vi "Update_Attribute_Tree_POLARIS.vi"(4 "Flush Tree?":bool, 5 "error in":errorcluster, 6 "Filter":string, 7 "Tree Control In":refnum<vi>, 8 "Camera Name In":T1 caption="Session In") -> (0 "error out":errorcluster, 2 "Tree Control Out":refnum<vi>, 3 "Session Out":T1)   [LabVIEW 2014]
doc: "The Update Attribute Tree subVI, enumerates the attributes available for the camera and populates the Attribute Tree control with the attribute list."
uses:
  <vilib>/userdefined/High Color/IMAQdx.ctl
  <vilib>/vision/driver/NI_Vision_Acquisition_Software.lvlib
  <resource>/objmgr/imaqdx.rc
panel:
  out "ValuesArray":string[](array[string])
  out "AttibuteArray":string[](array[string])
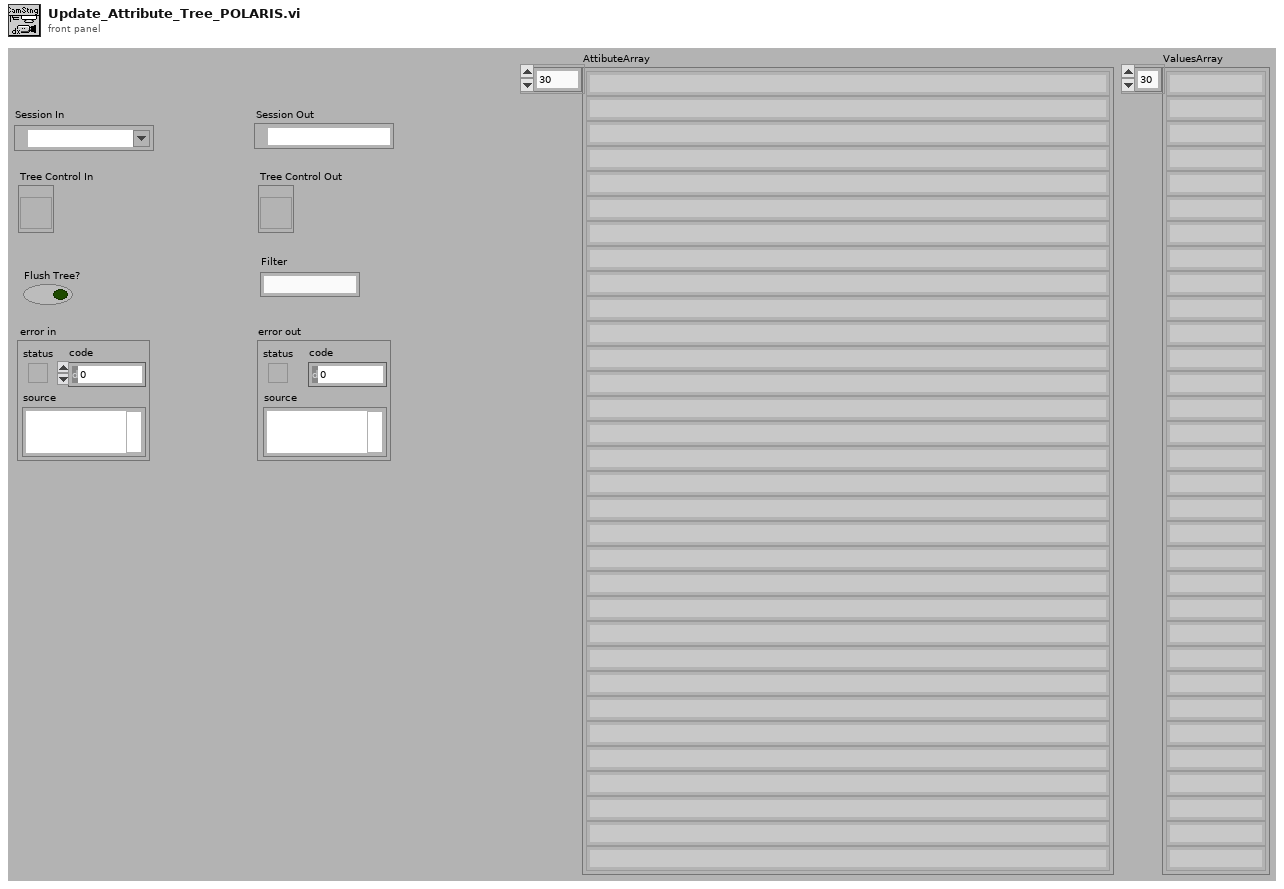
[diagram p1: front panel]
types:
  T1 = typedef "IMAQdx.ctl" = refnum<k21>
  T2 = typedef "NI_Vision_Acquisition_Software.lvlib/IMAQdx Attribute Type.ctl" = enum32{"U32", "I64", "DBL", "String", "Enum", "Bool", "Command"}
  T3 = cluster{"Attribute Type":T2, "Readable":bool, "Writable":bool, "Attribute Name":string}[]
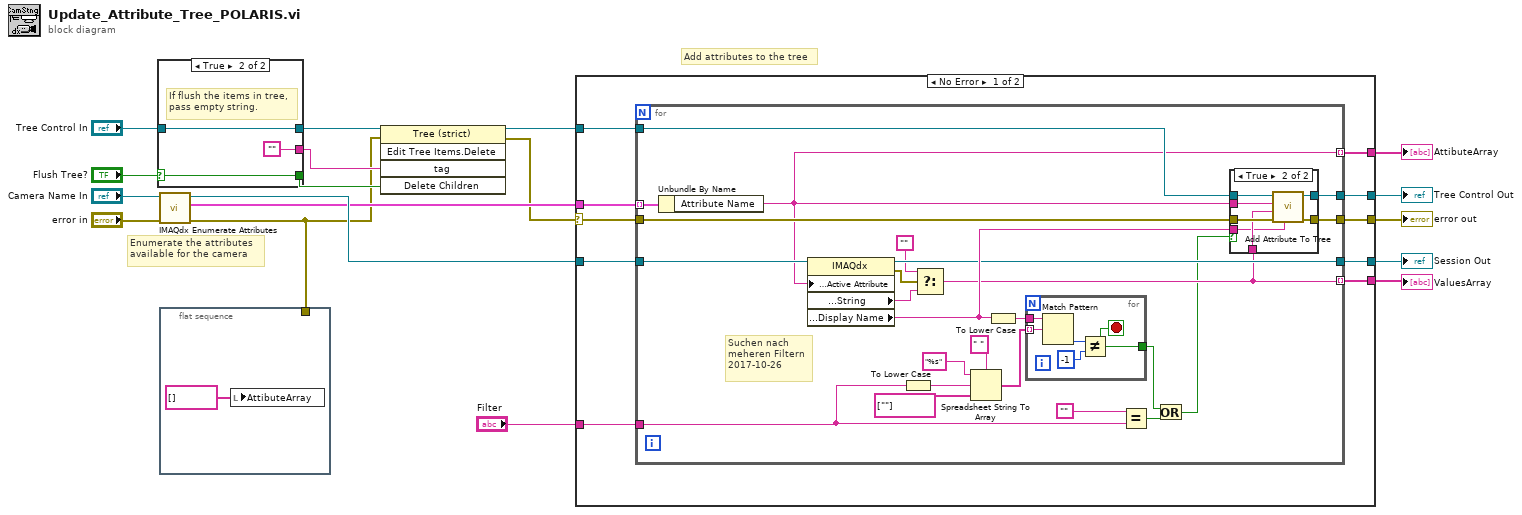
[diagram p0: block diagram]
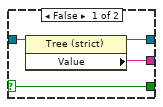
[diagram p2: hidden frame]
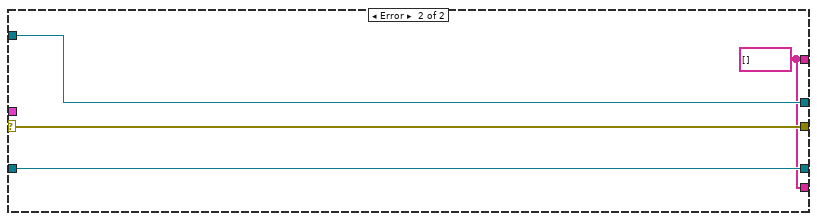
[diagram p4: hidden frame]
diagram:
  # "Add attributes to the tree"
  # "Enumerate the attributes \navailable for the camera"
  n1 = case shown="True" "Flush Tree?" {
    selector: "Flush Tree?" -> [w22 w25]
    tunnel: [w22 w25] -> w8
    tunnel: [w19 ""] -> w7
    tunnel: "Tree Control In" -> [w21 w23]
    tunnel: [w20 w23] -> w5
    frame False {
      n2 = property class="Tree (strict)"(reference=w21) -> (reference out=w20:refnum<vi>, "Value"=w19:string)  [unwired: 1 in, 1 out]
    }
    frame True {
      # "If flush the items in tree,\npass empty string."
    }
  }
  n3 = call <vilib>:"IMAQdx Enumerate Attributes.vi"("error in"="error in", "Session In"="Camera Name In") -> ("error out"=w3:errorcluster, "Attribute Information Array"=w17:T3, "Session Out"=w18:T1)  [unwired: 7 in]
  n4 = flat-sequence {
    tunnel: w3 -> [_]
    frame #0 {
      n5 = local write "AttibuteArray"(string[] []) -> ()
    }
  }
  n6 = invoke class="Tree (strict)" method="Edit Tree Items.Delete"(reference=w5, error in=w3, "tag"=w7, "Delete Children"=w8) -> (reference out=w12:refnum<vi>, error out=w11:errorcluster)  [unwired: 1 in, 3 out]
  n7 = case shown="No Error" w11 {
    selector: w11 -> [w34 w78]
    tunnel: w17 -> [w36 _]
    tunnel: w12 -> [w35 w76]
    tunnel: w18 -> [w33 w77]
    tunnel: [w32 w78] -> w10
    tunnel: [w31 w77] -> w14
    tunnel: [w30 w76] -> w13
    tunnel: [w29 w75] -> w4
    tunnel: [w28 w75] -> w2
    tunnel: "Filter" -> [w27 _]
    frame No Error {
      n8 = for {
        tunnel: w36 -> [w59] mode=indexing
        tunnel: w35 -> [w55]
        tunnel: w34 -> [w54]
        tunnel: w33 -> [w58]
        tunnel: [w57] -> w32
        tunnel: [w56] -> w31
        tunnel: [w53] -> w30
        tunnel: [w50] -> w29 mode=indexing
        tunnel: [w52] -> w28 mode=indexing
        tunnel: w27 -> [w42]
        # "Suchen nach \nmeheren Filtern\n2017-10-26"
        n9 = Unbundle By Name(w59) -> ("Attribute Name"=w50:string)
        n10 = property class="IMAQdx"(reference=w58, "Camera Attributes:Active Attribute"=w50) -> (reference out=w56:T1, error out=w47:errorcluster, "Camera Attributes:Value:String"=w45:string, "Camera Attributes:Display Name"=w60:string)  [unwired: 1 in]
        n11 = To Lower Case(string=w42) -> (all lower case string=w38:string)
        n12 = Select(t="", s=w47, f=w45) -> (s? t:f=w52:string)
        n13 = Spreadsheet String To Array(delimiter (Tab)=" ", format string="%s", spreadsheet string=w38, array type (2D Dbl)=string[] [""]) -> (array=w37:string[])
        n14 = To Lower Case(string=w60) -> (all lower case string=w43:string)
        n15 = for {
          tunnel: [w61] -> w48
          tunnel: w43 -> [w63]
          tunnel: w37 -> [w62] mode=indexing
          stop <- w61 stop-if-true
          n16 = Match Pattern(string=w63, regular expression=w62) -> (offset past match=w65:i32)  [unwired: 1 in, 3 out]
          n17 = Not Equal?(x=w65, y=-1) -> (x != y?=w61:bool)
        }
        n18 = Equal?(x="", y=w42) -> (x = y?=w49:bool)
        n19 = Or(x=w48, y=w49) -> (x .or. y?=w44:bool)
        n20 = case shown="True" w44 {
          tunnel: [w66 w74] -> w57
          tunnel: w55 -> [w67 w73]
          tunnel: w54 -> [w66 w72]
          tunnel: [w67 w71] -> w53
          tunnel: w52 -> [_ w70]
          tunnel: w50 -> [_ w69]
          tunnel: w60 -> [_ w68]
          frame False {
          }
          frame True {
            n21 = call "Add Attribute To Tree.vi"("Display Name"=w68, "error in"=w72, "Value"=w70, "Attribute Name"=w69, "Attribute Table In"=w73) -> ("error out"=w74:errorcluster, "Attribute Table Out"=w71:refnum<vi>)  [unwired: 5 in]
          }
        }
      }
    }
    frame Error {
      w75 = string[] []
    }
  }
  "error out" <- w10
  "Session Out" <- w14
  "Tree Control Out" <- w13
  "AttibuteArray" <- w4
  "ValuesArray" <- w2
